vi "loadOvenStatus.vi"() -> ()   [LabVIEW 2012]
uses:
  <vilib>/addons/database/Connection.llb/DB Tools Open Connec (Path).vi
  <vilib>/addons/database/Connection.llb/Conn Execute.vi
  <vilib>/addons/database/Recordset.llb/Rec Fetch Recordset Data (R).vi
  <vilib>/addons/database/Recordset.llb/Rec Destroy - Connection.vi
  <vilib>/addons/database/Recordset.llb/Rec Fetch Integer Data (R).vi
  <vilib>/addons/database/Recordset.llb/Rec Fetch Double Data (R).vi
  <vilib>/addons/database/_DB Variant To Data/Database Variant To Data.xnode
  <vilib>/addons/database/NI_Database_API.lvlib
panel:
  out "data":dbl format="%.2f"
  out "concatenated string 4":string
  out "concatenated string 3":string
  out "error out 2":errorcluster
  out "data 9":string
  out "data 8":string
  out "concatenated string 2":string
  out "before substring 2":string
  out "data 7":string
  out "recordset data":variant[][](array[variant])
  out "substring 2":string
  out "AsciiOutput":string
  out "concatenated string":string
  out "error out":errorcluster
  out "String":string
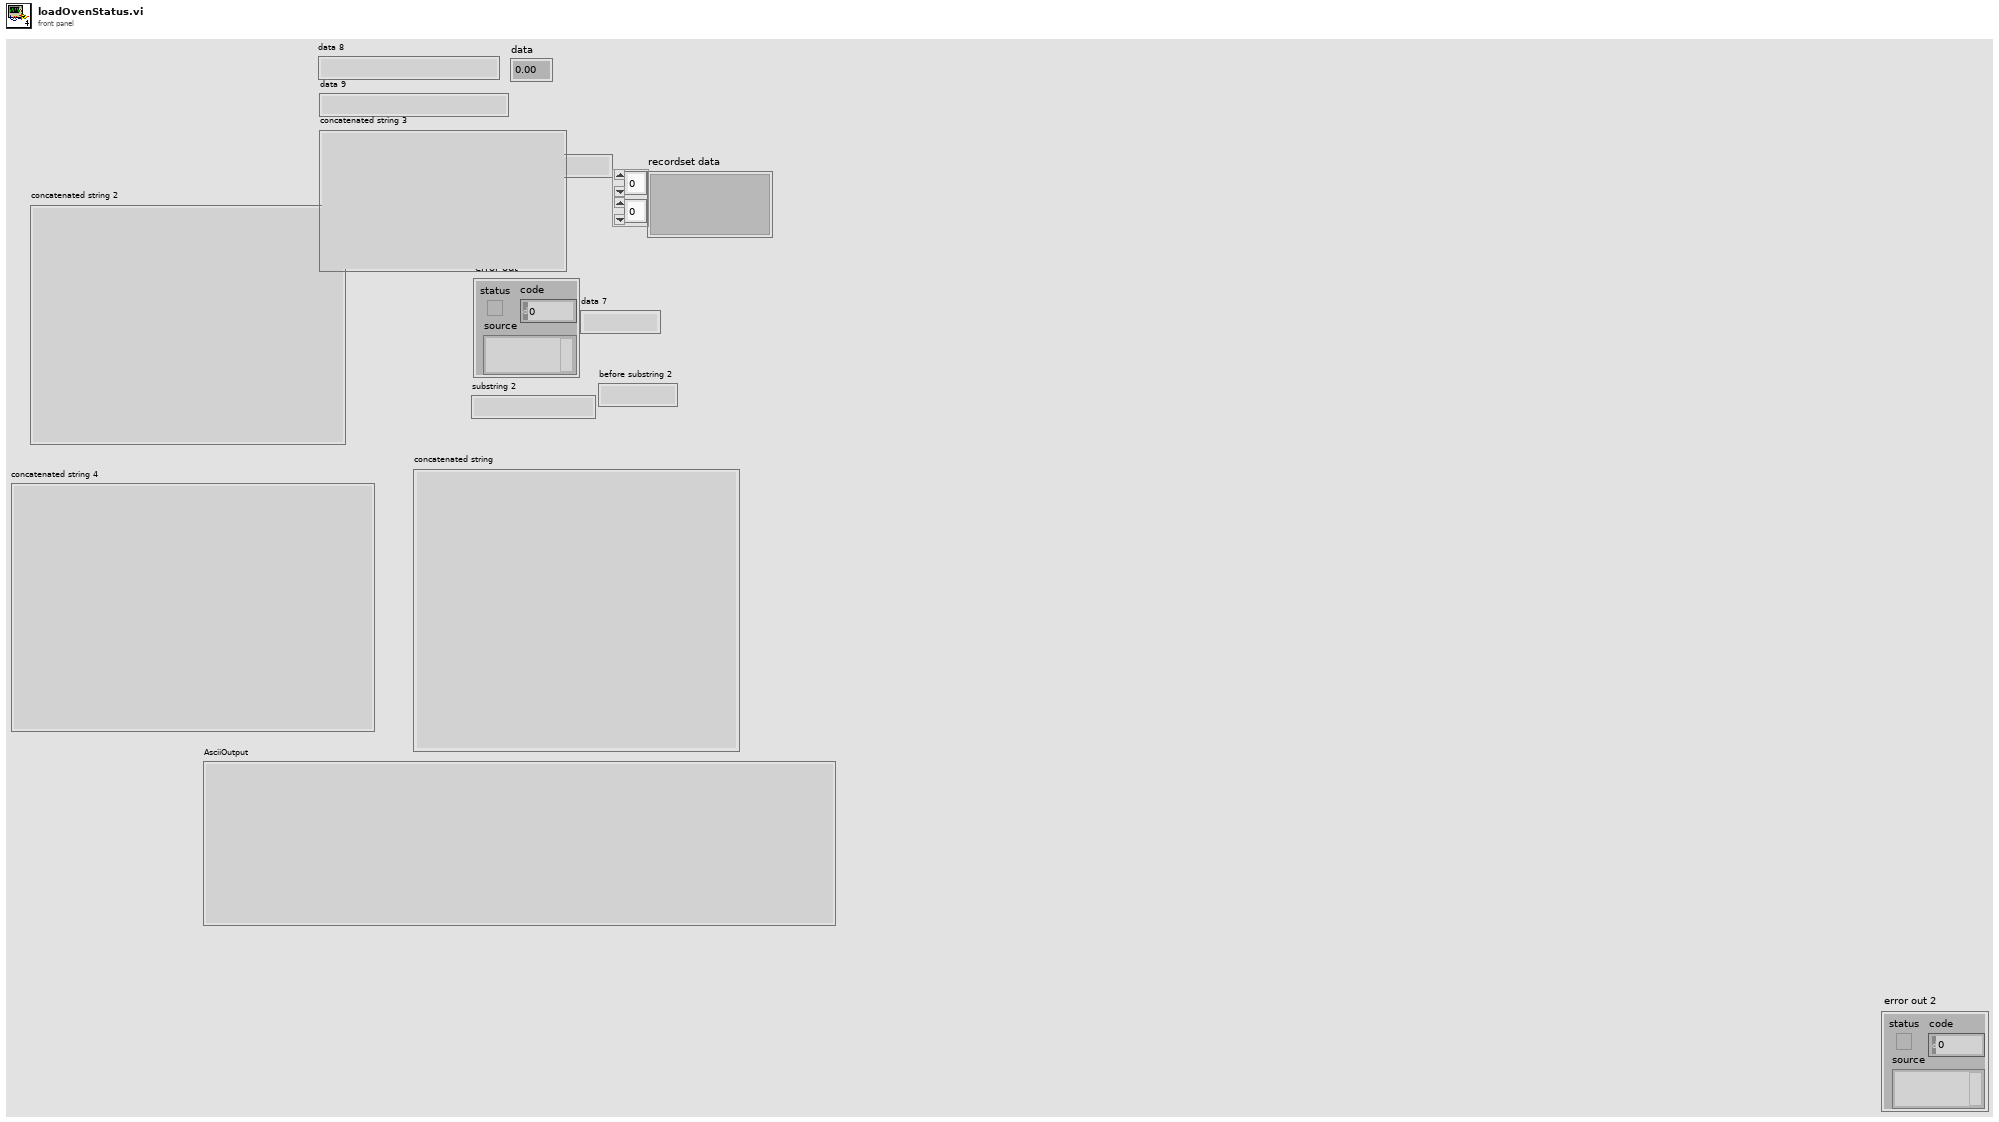
[diagram p1: front panel]
types:
  T1 = typedef "NI_Database_API.lvlib/Conn ObjectReference.ctl" = refnum<k1>
  T2 = typedef "NI_Database_API.lvlib/Rec ObjectReference.ctl" = refnum<k1>
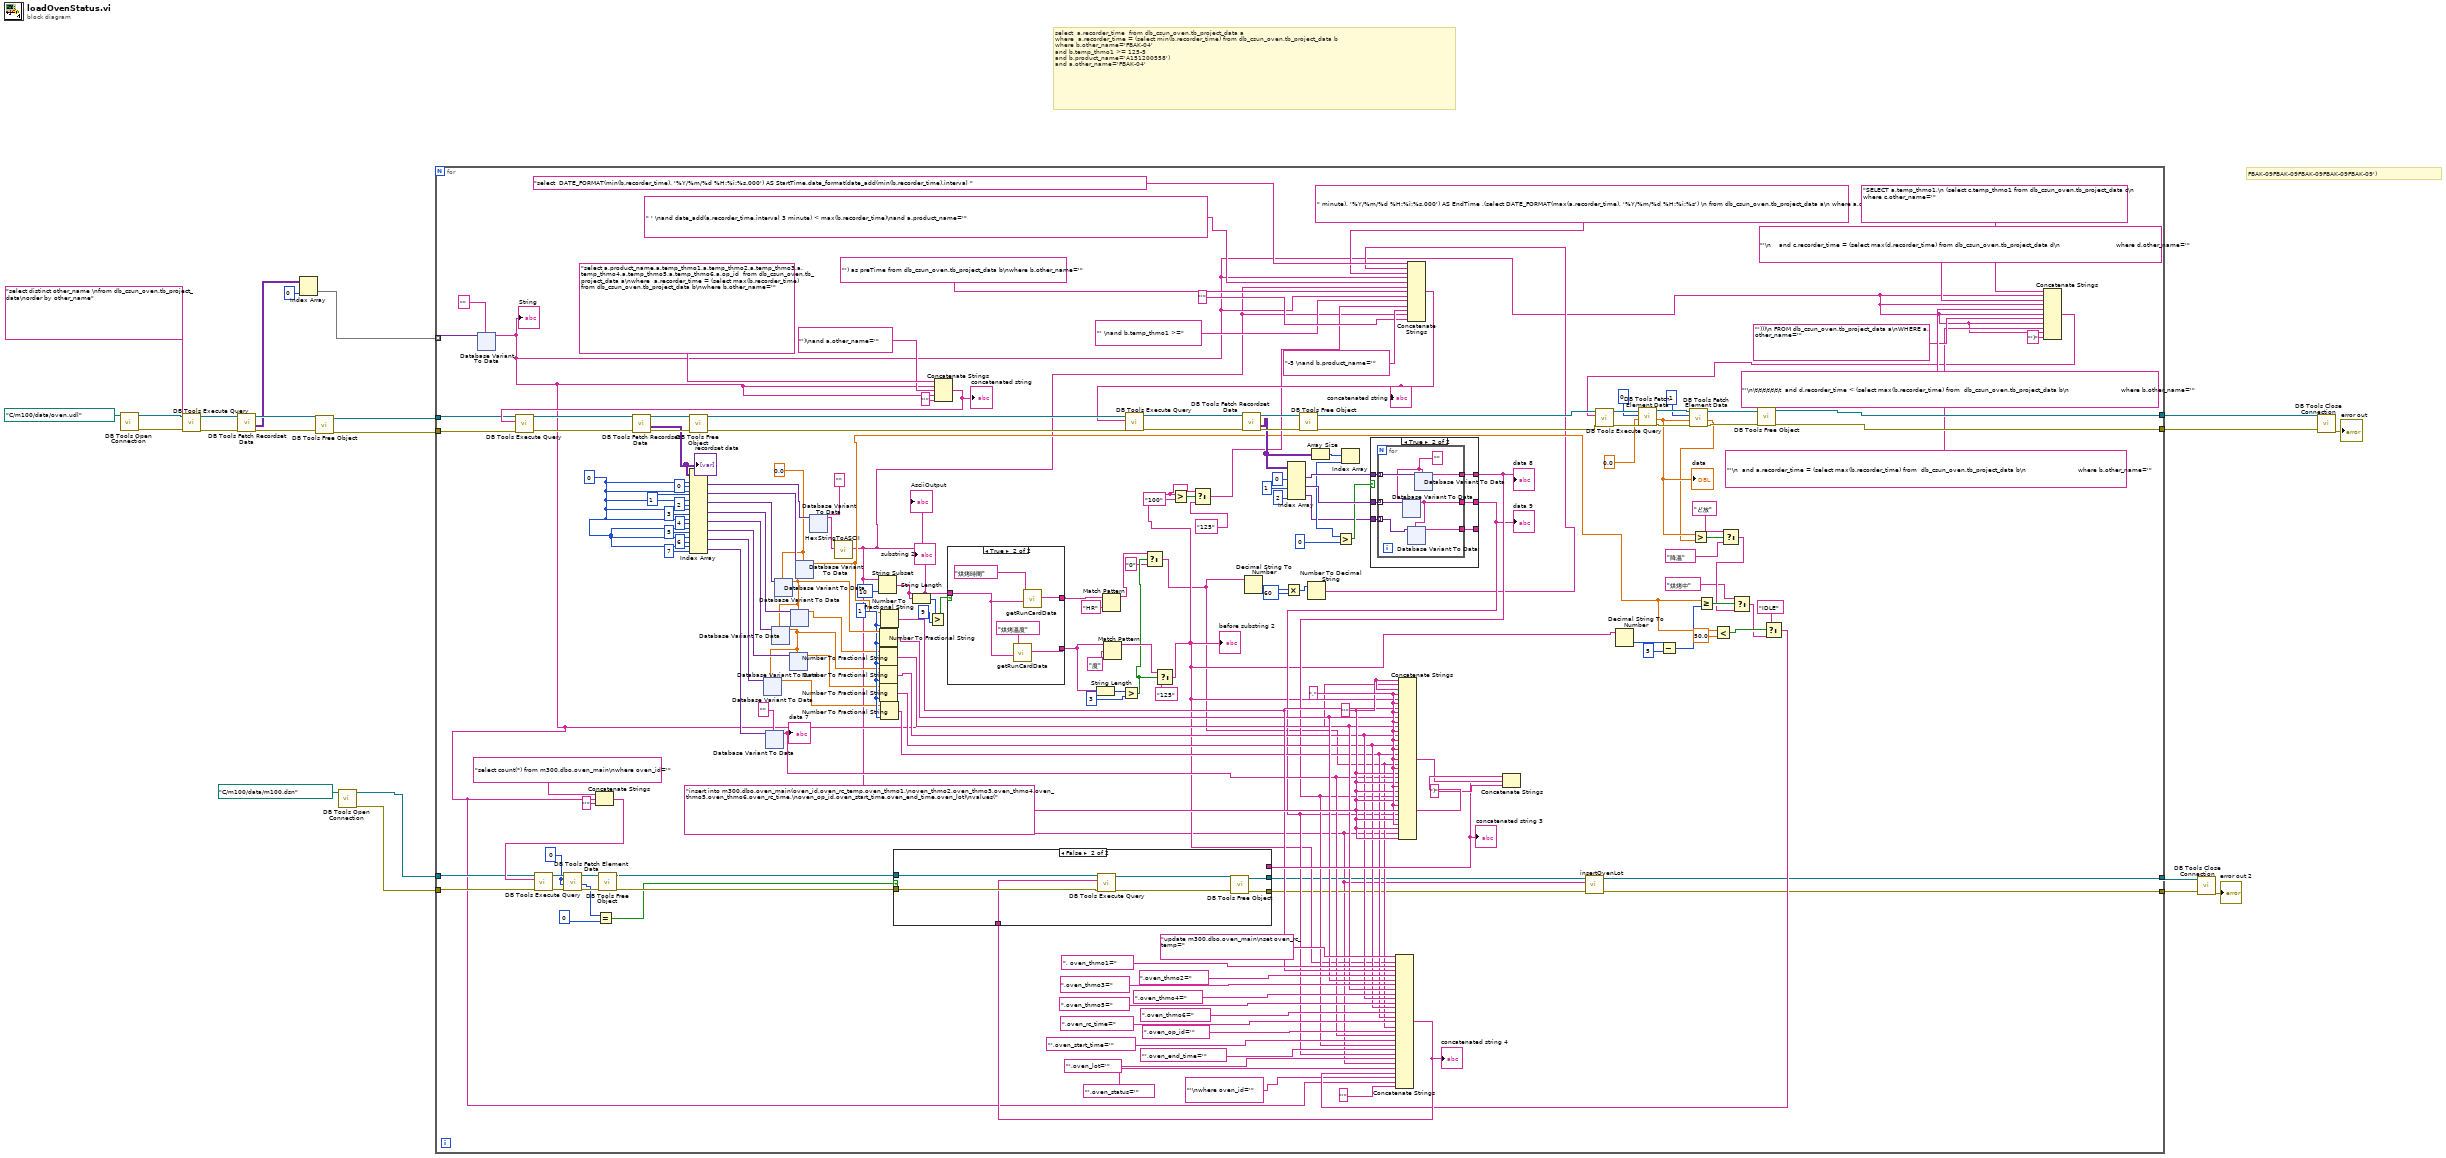
[diagram p0: block diagram]
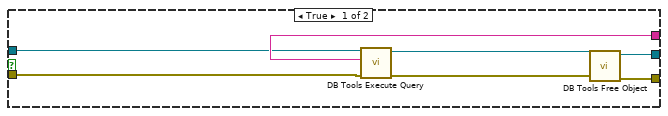
[diagram p2: hidden frame]
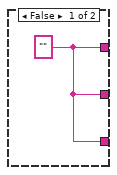
[diagram p3: hidden frame]
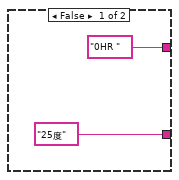
[diagram p4: hidden frame]
diagram:
  # "FBAK-09FBAK-09FBAK-09FBAK-09FBAK-09')"
  # "select  a.recorder_time  from db_csun_oven.tb_project_data a\nwhere  a.recorder_time = (select min(b.recorder_time) from db_csun_oven.tb_project_data b\nwhere b.other_name='FBAK-04' \nand b.temp_thmo1 >= 125-5\nand b.product_name='A151200558')\nand a.other_name='FBAK-04'"
  n1 = call-poly <vilib>:"DB Tools Open Connection.vi"("connection information"=path "C:/m100/data/oven.udl") -> ("error out"=w16:errorcluster, "connection reference"=w20:T1)  [unwired: 7 in]
  n2 = call-poly <vilib>:"DB Tools Execute Query.vi"("error in (no error)"=w16, "SQL query"="select distinct other_name \nfrom db_csun_oven.tb_project_data\norder by other_name", "connection reference"=w20) -> ("error out"=w15:errorcluster, "recordset reference"=w19:T2)  [unwired: 5 in]
  n3 = call-poly <vilib>:"DB Tools Fetch Recordset Data.vi"("error in (no error)"=w15, "recordset reference"=w19) -> ("error out"=w14:errorcluster, "recordset data"=w11:variant[][], "recordset reference out"=w18:T2)  [unwired: 3 in]
  n4 = Index Array(array=w11, index (col)=0 ("disabled index (col)")) -> (element=w9:variant[])  [unwired: 1 in]
  n5 = call-poly <vilib>:"DB Tools Free Object.vi"("error in (no error)"=w14, "recordset reference"=w18) -> ("error out"=w13:errorcluster, "connection reference"=w17:T1)  [unwired: 8 in]
  n6 = call-poly <vilib>:"DB Tools Open Connection.vi"("connection information"=path "C:/m100/data/m100.dsn") -> ("error out"=w5:errorcluster, "connection reference"=w4:T1)  [unwired: 7 in]
  n7 = for {
    tunnel: w9 -> [w183] mode=indexing
    tunnel: w13 -> [w202]
    tunnel: w17 -> [w184]
    tunnel: [w77] -> w8
    tunnel: [w74] -> w7
    tunnel: w4 -> [w119]
    tunnel: w5 -> [w118]
    tunnel: [w25] -> w2
    tunnel: [w24] -> w1
    w115 = 0
    w123 = "'" ("string")
    w129 = i16 1 ("precision (6)")
    w124 = "," ("string")
    w169 = 0.0
    w168 = 0 ("disabled index (row)")
    n8 = xnode "Database Variant To Data"("database variant"=w183, "type"="") -> ("data"=w37:string)  [unwired: 1 in, 1 out]
    "String" <- w37
    n9 = Concatenate Strings("select count(*) from m300.dbo.oven_main\nwhere oven_id='" ("string"), w37, "'" ("string")) -> (w120:string)
    n10 = call-poly <vilib>:"DB Tools Execute Query.vi"("error in (no error)"=w118, "SQL query"=w120, "connection reference"=w119) -> ("error out"=w117:errorcluster, "recordset reference"=w116:T2)  [unwired: 5 in]
    n11 = call-poly <vilib>:"DB Tools Fetch Element Data.vi"("error in (no error)"=w117, "type"=w115, "column index"=w115, "recordset reference"=w116) -> ("error out"=w113:errorcluster, "data"=w112:i32, "recordset reference out"=w114:T2)  [unwired: 3 in]
    n12 = Equal?(x=w112, y=0 ("data")) -> (x = y?=w109:bool)
    n13 = call-poly <vilib>:"DB Tools Free Object.vi"("error in (no error)"=w113, "recordset reference"=w114) -> ("error out"=w110:errorcluster, "connection reference"=w111:T1)  [unwired: 8 in]
    n14 = Concatenate Strings("select a.product_name,a.temp_thmo1,a.temp_thmo2,a.temp_thmo3,a.temp_thmo4,a.temp_thmo5,a.temp_thmo6,a.op_id  from db_csun_oven.tb_project_data a\nwhere  a.recorder_time = (select max(b.recorder_time) from db_csun_oven.tb_project_data b\nwhere b.other_name='", w37, "')\nand a.other_name='" ("string"), w37, "'" ("string")) -> (w194:string)
    "concatenated string" <- w194
    n15 = call-poly <vilib>:"DB Tools Execute Query.vi"("error in (no error)"=w202, "SQL query"=w194, "connection reference"=w184) -> ("error out"=w200:errorcluster, "recordset reference"=w201:T2)  [unwired: 5 in]
    n16 = call-poly <vilib>:"DB Tools Fetch Recordset Data.vi"("error in (no error)"=w200, "recordset reference"=w201) -> ("error out"=w198:errorcluster, "recordset data"=w193:variant[][], "recordset reference out"=w199:T2)  [unwired: 3 in]
    "recordset data" <- w193
    n17 = call-poly <vilib>:"DB Tools Free Object.vi"("error in (no error)"=w198, "recordset reference"=w199) -> ("error out"=w156:errorcluster, "connection reference"=w157:T1)  [unwired: 8 in]
    n18 = Index Array(array=w193, index (row) #1=w168, index (col) #1=0 ("disabled index (col)"), index (row) #2=w168, index (col) #2=1 ("disabled index (col)"), index (row) #3=w168, index (col) #3=2 ("index (col)"), index (row) #4=w168, index (col) #4=3 ("index (col)"), index (row) #5=w168, index (col) #5=4 ("index (col)"), index (row) #6=w168, index (col) #6=5 ("index (col)"), index (row) #7=w168, index (col) #7=6 ("index (col)"), index (row) #8=w168, index (col) #8=7 ("disabled index (col)")) -> (element #1=w181:variant, element #2=w175:variant, element #3=w174:variant, element #4=w173:variant, element #5=w172:variant, element #6=w171:variant, element #7=w170:variant, element #8=w166:variant)
    n19 = xnode "Database Variant To Data"("database variant"=w166, "type"="") -> ("data"=w93:string)  [unwired: 1 in, 1 out]
    "data 7" <- w93
    n20 = xnode "Database Variant To Data"("database variant"=w174, "type"=w169) -> ("data"=w135:dbl)  [unwired: 1 in, 1 out]
    n21 = xnode "Database Variant To Data"("database variant"=w172, "type"=w135) -> ("data"=w127:dbl)  [unwired: 1 in, 1 out]
    n22 = xnode "Database Variant To Data"("database variant"=w170, "type"=w127) -> ("data"=w125:dbl)  [unwired: 1 in, 1 out]
    n23 = xnode "Database Variant To Data"("database variant"=w171, "type"=w127) -> ("data"=w126:dbl)  [unwired: 1 in, 1 out]
    n24 = xnode "Database Variant To Data"("database variant"=w173, "type"=w135) -> ("data"=w128:dbl)  [unwired: 1 in, 1 out]
    n25 = xnode "Database Variant To Data"("database variant"=w175, "type"=w169) -> ("data"=w62:dbl)  [unwired: 1 in, 1 out]
    n26 = xnode "Database Variant To Data"("database variant"=w181, "type"="") -> ("data"=w154:string)  [unwired: 1 in, 1 out]
    n27 = call "HexStringToASCII.vi"("HexIStringnput"=w154) -> ("AsciiOutput"=w23:string)  [unwired: 10 in]
    "AsciiOutput" <- w23
    n28 = String Subset(string=w23, length (rest)=10 ("length (rest)")) -> (substring=w188:string)  [unwired: 1 in]
    "substring 2" <- w188
    n29 = Number To Fractional String(number=w135, precision (6)=w129) -> (F-format string=w104:string)  [unwired: 2 in]
    n30 = Number To Fractional String(number=w128, precision (6)=w129) -> (F-format string=w102:string)  [unwired: 2 in]
    n31 = Number To Fractional String(number=w127, precision (6)=w129) -> (F-format string=w100:string)  [unwired: 2 in]
    n32 = Number To Fractional String(number=w126, precision (6)=w129) -> (F-format string=w98:string)  [unwired: 2 in]
    n33 = Number To Fractional String(number=w62, precision (6)=w129) -> (F-format string=w106:string)  [unwired: 2 in]
    n34 = Number To Fractional String(number=w125, precision (6)=w129) -> (F-format string=w96:string)  [unwired: 2 in]
    n35 = String Length(string=w188) -> (length=w187:i32)
    n36 = Greater?(x=w187, y=9) -> (0:w185:bool)
    n37 = case shown="True" w185 {
      tunnel: w188 -> [_ w587]
      tunnel: ["0HR " ("data") w588] -> w164
      tunnel: ["25度" ("data") w585] -> w53
      frame False {
      }
      frame True {
        n38 = call "getRunCardData.vi"("Jobno"=w587, "RCName"="烘烤溫度") -> ("data"=w585:string)  [unwired: 8 in, 1 out]
        n39 = call "getRunCardData.vi"("Jobno"=w587, "RCName"="烘烤時間") -> ("data"=w588:string)  [unwired: 8 in, 1 out]
      }
    }
    n40 = String Length(string=w53) -> (length=w52:i32)
    n41 = Match Pattern(string=w164, regular expression="HR") -> (before substring=w47:string)  [unwired: 1 in, 3 out]
    n42 = Match Pattern(string=w53, regular expression="度") -> (before substring=w50:string)  [unwired: 1 in, 3 out]
    n43 = Greater?(x=w52, y=3) -> (0:w45:bool)
    n44 = Select(t=w47, s=w45, f="0") -> (s? t:f=w46:string)
    n45 = Select(t=w50, s=w45, f="125") -> (s? t:f=w49:string)
    "before substring 2" <- w49
    n46 = Greater?(x=w49, y="100") -> (0:w138:bool)
    n47 = Select(t=w49, s=w138, f="125" ("t")) -> (s? t:f=w137:string)
    n48 = Decimal String To Number(string=w46) -> (number=w134:i32)  [unwired: 2 in, 1 out]
    n49 = Multiply(x=w134, y=60) -> (x*y=w149:i32)
    n50 = Number To Decimal String(number=w149) -> (decimal integer string=w43:string)  [unwired: 1 in]
    n51 = Concatenate Strings("select  DATE_FORMAT(min(b.recorder_time), '%Y/%m/%d %H:%i:%s.000') AS StartTime,date_format(date_add(min(b.recorder_time),interval " ("string"), w43, " minute), '%Y/%m/%d %H:%i:%s.000') AS EndTime ,(select DATE_FORMAT(max(a.recorder_time), '%Y/%m/%d %H:%i:%s') \n from db_csun_oven.tb_project_data a\n where a.other_name='", w37, " ' \nand date_add(a.recorder_time,interval 3 minute) < max(b.recorder_time)\nand a.product_name='", w23, "') as preTime from db_csun_oven.tb_project_data b\nwhere b.other_name='", w37, "' \nand b.temp_thmo1 >=" ("string"), w137, "-5 \nand b.product_name='" ("string"), w23, "'" ("string")) -> (w155:string)
    "concatenated string 2" <- w155
    n52 = call-poly <vilib>:"DB Tools Execute Query.vi"("error in (no error)"=w156, "SQL query"=w155, "connection reference"=w157) -> ("error out"=w160:errorcluster, "recordset reference"=w161:T2)  [unwired: 5 in]
    n53 = call-poly <vilib>:"DB Tools Fetch Recordset Data.vi"("error in (no error)"=w160, "recordset reference"=w161) -> ("error out"=w158:errorcluster, "recordset data"=w144:variant[][], "recordset reference out"=w159:T2)  [unwired: 3 in]
    n54 = Index Array(array=w144, index (col) #1=0 ("disabled index (col)"), index (col) #2=1 ("disabled index (col)"), index (col) #3=2 ("index (col)")) -> (element #1=w146:variant[], element #2=w145:variant[], element #3=w80:variant[])  [unwired: 3 in]
    n55 = call-poly <vilib>:"DB Tools Free Object.vi"("error in (no error)"=w158, "recordset reference"=w159) -> ("error out"=w76:errorcluster, "connection reference"=w79:T1)  [unwired: 8 in]
    n56 = Array Size(array=w144) -> (size(s)=w143:i32[])
    n57 = Index Array(array=w143) -> (element=w142:i32)  [unwired: 1 in]
    n58 = Greater?(x=w142, y=0) -> (0:w140:bool)
    n59 = case shown="True" w140 {
      tunnel: w146 -> [_ w223]
      tunnel: w145 -> [_ w222]
      tunnel: [w217 w221] -> w91
      tunnel: [w217 w220] -> w89
      tunnel: w80 -> [_ w219]
      tunnel: [w217 w218] -> _
      frame False {
        w217 = ""
      }
      frame True {
        n60 = for {
          tunnel: w223 -> [w230] mode=indexing
          tunnel: w222 -> [w229] mode=indexing
          tunnel: [w227] -> w221
          tunnel: [w225] -> w220
          tunnel: w219 -> [w226] mode=indexing
          tunnel: [w224] -> w218
          w228 = ""
          n61 = xnode "Database Variant To Data"("database variant"=w229, "type"=w228) -> ("data"=w225:string)  [unwired: 1 in, 1 out]
          n62 = xnode "Database Variant To Data"("database variant"=w226, "type"=w225) -> ("data"=w224:string)  [unwired: 1 in, 1 out]
          n63 = xnode "Database Variant To Data"("database variant"=w230, "type"=w228) -> ("data"=w227:string)  [unwired: 1 in, 1 out]
        }
      }
    }
    "data 8" <- w91
    "data 9" <- w89
    n64 = Concatenate Strings(w123, w37, w123, w124, w49, w124, w106, w124, w104, w124, w102, w124, w100, w124, w98, w124, w96, w124, w46, w124, w123, w93, w123, w124, w123, w91, w123, w124, w123, w89, w123, w124, w123, w23, w123) -> (w132:string)
    n65 = Concatenate Strings("insert into m300.dbo.oven_main(oven_id,oven_rc_temp,oven_thmo1,\noven_thmo2,oven_thmo3,oven_thmo4,oven_thmo5,oven_thmo6,oven_rc_time,\noven_op_id,oven_start_time,oven_end_time,oven_lot)\nvalues(", w132, ")" ("string")) -> (w130:string)
    "concatenated string 3" <- w130
    n66 = Decimal String To Number(string=w49) -> (number=w68:i32)  [unwired: 2 in, 1 out]
    n67 = Subtract(x=w68, y=5) -> (x-y=w66:i32)
    n68 = Greater Or Equal?(x=w62, y=w66) -> (x >= y?=w65:bool)
    n69 = Less?(x=w62, y=50.0) -> (x < y?=w60:bool)
    n70 = Concatenate Strings("SELECT a.temp_thmo1,\n (select c.temp_thmo1 from db_csun_oven.tb_project_data c\n  where c.other_name='", w37, "'\n    and c.recorder_time = (select max(d.recorder_time) from db_csun_oven.tb_project_data d\n                            where d.other_name='" ("string"), w37, "'\n\t\t\t\t\t\t\t  and d.recorder_time < (select max(b.recorder_time) from  db_csun_oven.tb_project_data b\n                          where b.other_name='" ("string"), w37, "')))\n FROM db_csun_oven.tb_project_data a\nWHERE a.other_name='" ("string"), w37, "'\n  and a.recorder_time = (select max(b.recorder_time) from  db_csun_oven.tb_project_data b\n                          where b.other_name='" ("string"), w37, "')" ("string")) -> (w35:string)
    n71 = call-poly <vilib>:"DB Tools Execute Query.vi"("error in (no error)"=w76, "SQL query"=w35, "connection reference"=w79) -> ("error out"=w75:errorcluster, "recordset reference"=w78:T2)  [unwired: 5 in]
    n72 = call-poly <vilib>:"DB Tools Fetch Element Data.vi"("error in (no error)"=w75, "type"=0.0, "column index"=0, "recordset reference"=w78) -> ("error out"=w31:errorcluster, "data"=w29:dbl, "recordset reference out"=w34:T2)  [unwired: 3 in]
    "data" <- w29
    n73 = call-poly <vilib>:"DB Tools Fetch Element Data.vi"("error in (no error)"=w31, "type"=w29, "column index"=1, "recordset reference"=w34) -> ("error out"=w32:errorcluster, "data"=w28:dbl, "recordset reference out"=w33:T2)  [unwired: 3 in]
    n74 = Greater?(x=w29, y=w28) -> (0:w71:bool)
    n75 = Select(t="ど放", s=w71, f="降溫") -> (s? t:f=w64:string)
    n76 = Select(t="烘烤中", s=w65, f=w64) -> (s? t:f=w59:string)
    n77 = call-poly <vilib>:"DB Tools Free Object.vi"("error in (no error)"=w32, "recordset reference"=w33) -> ("error out"=w74:errorcluster, "connection reference"=w77:T1)  [unwired: 8 in]
    n78 = Select(t="IDLE", s=w60, f=w59) -> (s? t:f=w55:string)
    n79 = Concatenate Strings("update m300.dbo.oven_main\nset oven_rc_temp=" ("string"), w49, ", oven_thmo1=" ("string"), w106, ",oven_thmo2=" ("string"), w104, ",oven_thmo3=" ("string"), w102, ",oven_thmo4=" ("string"), w100, ",oven_thmo5=" ("string"), w98, ",oven_thmo6=" ("string"), w96, ",oven_rc_time=" ("string"), w46, ",oven_op_id='" ("string"), w93, "',oven_start_time='" ("string"), w91, "',oven_end_time='" ("string"), w89, "',oven_lot='" ("string"), w23, "',oven_status='" ("string"), w55, "'\nwhere oven_id='" ("string"), w37, "'" ("string")) -> (w87:string)
    "concatenated string 4" <- w87
    n80 = case shown="False" w109 {
      tunnel: w130 -> [w207 _]
      tunnel: [w206 w214] -> w26
      tunnel: [w205 w213] -> w27
      tunnel: w111 -> [w204 w212]
      tunnel: w110 -> [w203 w211]
      tunnel: w87 -> [_ w210]
      frame True {
        n81 = call-poly <vilib>:"DB Tools Execute Query.vi"("error in (no error)"=w203, "SQL query"=w207, "connection reference"=w204) -> ("error out"=w208:errorcluster, "recordset reference"=w209:T2)  [unwired: 5 in]
        n82 = call-poly <vilib>:"DB Tools Free Object.vi"("error in (no error)"=w208, "recordset reference"=w209) -> ("error out"=w205:errorcluster, "connection reference"=w206:T1)  [unwired: 8 in]
      }
      frame False {
        n83 = call-poly <vilib>:"DB Tools Execute Query.vi"("error in (no error)"=w211, "SQL query"=w210, "connection reference"=w212) -> ("error out"=w215:errorcluster, "recordset reference"=w216:T2)  [unwired: 5 in]
        n84 = call-poly <vilib>:"DB Tools Free Object.vi"("error in (no error)"=w215, "recordset reference"=w216) -> ("error out"=w213:errorcluster, "connection reference"=w214:T1)  [unwired: 8 in]
      }
    }
    n85 = call "insertOvenLot.vi"("error in (no error)"=w27, "lot list"=w23, "connection reference"=w26) -> ("error out"=w24:errorcluster, "connection reference out"=w25:T1)  [unwired: 7 in]
  }
  n86 = call <vilib>:"DB Tools Close Connection.vi"("error in (no error)"=w1, "connection reference"=w2) -> ("error out"=→"error out 2":errorcluster)  [unwired: 5 in]
  n87 = call <vilib>:"DB Tools Close Connection.vi"("error in (no error)"=w7, "connection reference"=w8) -> ("error out"=→"error out":errorcluster)  [unwired: 5 in]
